vi "create Timings.vi"(8 "error in (no error)":errorcluster, 10 "Parameters":u32[](array[numeric]), 11 "HF-Felder in":refnum<class "HF-Felder.lvclass">) -> (0 "error out":errorcluster, 1 "wait":i32[](array[numeric]), 2 "timeout":u32[](array[numeric]), 3 "HF-Felder out":refnum<class "HF-Felder.lvclass">)   [LabVIEW 2013, in "HF-Felder.lvclass"]
uses:
  HF-Felder.lvclass
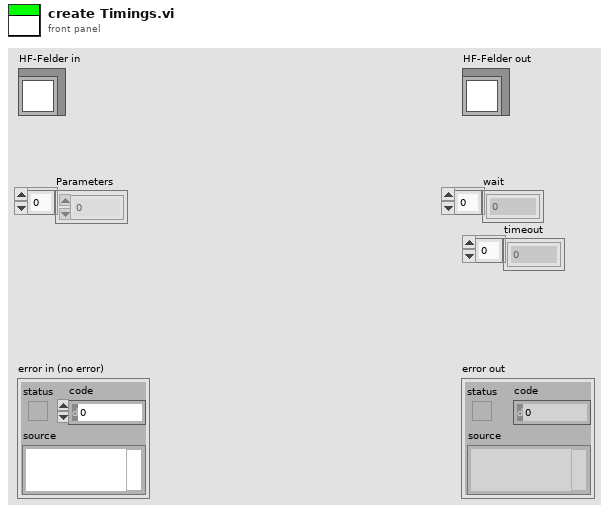
[diagram p1: front panel]
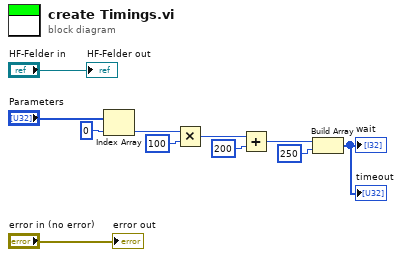
[diagram p0: block diagram]
diagram:
  n1 = Index Array(array="Parameters", index=0) -> (element=w9:u32)
  n2 = Multiply(x=w9, y=u32 100) -> (x*y=w3:u32)
  n3 = Add(x=w3, y=u32 200) -> (x+y=w1:u32)
  n4 = Build Array(w1, u32 250 ("element")) -> (→"timeout" →"wait":u32[])
  "error out" <- "error in (no error)"
  "HF-Felder out" <- "HF-Felder in"
